vi "Watchdog (TESTER).vi"() -> ()   [LabVIEW 2019]
uses:
  <vilib>/RTwatchdog.llb/Watchdog expiration actions.ctl
  <vilib>/RTwatchdog.llb/Watchdog status enum.ctl
panel:
  in  "Expire Watchdog":bool
  in  "Stop":bool
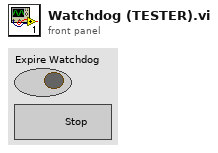
[diagram p1: front panel]
types:
  T1 = typedef "Watchdog expiration actions.ctl" = cluster{"reset system":bool, "restart LabVIEW Runtime":bool, "occurrence":bool, "trigger protocol":enum16{"active high", "active low", "open collector"}, "trigger line":enum16{"none", "line 0", "line 1", "line 2", "line 3", "line 4", "line 5", "line 6", "line 7", "SMB line 0"}, "disable watchdog on VI exit":bool}
  T2 = typedef "Watchdog status enum.ctl" = enum16{"disabled", "expired", "running"}
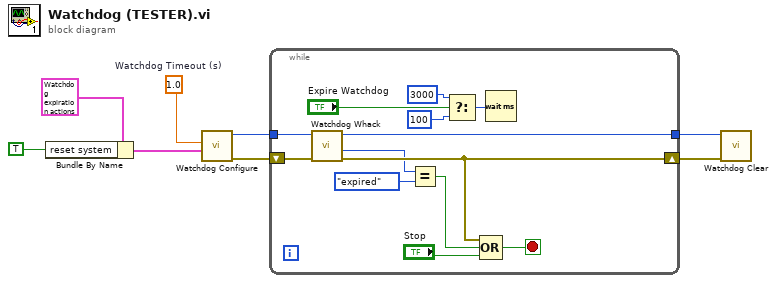
[diagram p0: block diagram]
diagram:
  w4 = 1.0  # Watchdog Timeout (s)
  n1 = Bundle By Name(cluster=T1 {"reset system"=FALSE, "restart LabVIEW Runtime"=FALSE, "occurrence"=FALSE, "trigger protocol"=enum."active high", "trigger line"=enum."none", "disable watchdog on VI exit"=TRUE} ("expiration actions"), "reset system"=TRUE) -> (w3:T1)
  n2 = call <vilib>:"Watchdog Configure.vi"("expiration actions"=w3, "timeout (1 sec)"=w4) -> ("error out"=w6:errorcluster, "watchdogID"=w5:u64)  [unwired: 2 in, 2 out]
  n3 = while {
    tunnel: [w19] -> w7
    tunnel: w5 -> [w20]
    shift-right: [w13] -> w8
    shift-left: w6 -> [w21]
    stop <- w14 stop-if-true
    n4 = call <vilib>:"Watchdog Whack.vi"("error in (no error)"=w21, "watchdogID in"=w20) -> ("error out"=w13:errorcluster, "watchdog status"=w12:T2, "watchdogID out"=w19:u64)  [unwired: 3 in]
    n5 = Equal?(x=w12, y=Watchdog_status_enum."expired") -> (x = y?=w9:bool)
    n6 = Select(t=u32 3000 ("wait (msec)"), s="Expire Watchdog", f=u32 100 ("wait (msec)")) -> (s? t:f=w18:u32)
    n7 = Compound Arithmetic op=OR(w13, w9, "Stop") -> (w14:bool)
    n8 = Wait (ms)(milliseconds to wait=w18) -> ()  [unwired: 1 out]
  }
  n9 = call <vilib>:"Watchdog Clear.vi"("error in (no error)"=w8, "watchdogID in"=w7) -> ()  [unwired: 5 in, 1 out]
